vi "Flicker Main.vi"(8 "error in (no error)":errorcluster, 11 "Master":refnum<queue>) -> (0 "error out":errorcluster)   [LabVIEW 2014, in "Flicker.lvlib"]
doc: "This VI provides control and an interface for the photometric flicker measurements. It is built based on the queued message handler template and low level function VI's developed at CLTC. It is made to function as a stand-alone piece of sofware, or to be controlled by the Measurement Control package."
uses:
  Flicker.lvlib
  support/Message Queue/Message Cluster.ctl
  Settings/Settings.ctl
  Acquisition/Hardware Configuration.ctl
  Acquisition/Signal Type.ctl
  Logging/Logging Configuration.ctl
  controls/Flicker UI Data.ctl
  support/Message Queue/Enqueue Message (Single).vi
  support/Message Queue/Enqueue Message (Array).vi
  <vilib>/Utility/error.llb/Error Cluster From Error Code.vi
  <vilib>/ErrorRing/Error Ring.xnode
  Acquisition/Flicker Acquisition.lvlib
  Logging/Flicker Logging.lvlib
  Settings/Flicker Settings.lvlib
  support/User Event - Stop/Flicker User Event - Stop.lvlib
  support/Message Queue/Flicker Message Queue.lvlib
panel:
  out "Data":waveform(dbl)[](graph)
  in  "Settings":bool
  in  "Start Acquisition":bool
  in  "Stop":bool
  out "Status":string
  in  "Exit":bool
  # "Flicker"
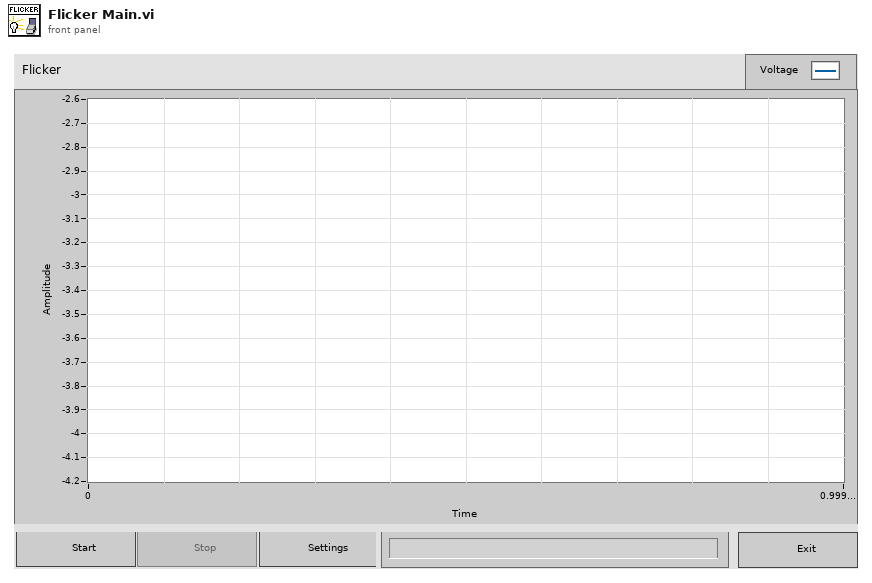
[diagram p1: front panel]
types:
  T1 = typedef "Flicker.lvlib/Flicker UI Data.ctl" = cluster{"Start Ref":refnum<vi>, "Stop Ref":refnum<vi>, "Settings Ref":refnum<vi>, "Exit Ref":refnum<vi>, "Status Ref":refnum<vi>, "WFGraph Refnum":refnum<vi>}
  T2 = typedef "Flicker.lvlib/Flicker Settings.lvlib/Settings.ctl" = cluster{"Hardware Configuration":T3, "Logging Configuration":T5}
  T3 = typedef "Flicker.lvlib/Flicker Acquisition.lvlib/Hardware Configuration.ctl" = cluster{"DAQmx Task Name":refnum<k21>, "HW Refnum <Replace Me>":string, "Signal Type <Replace Me>":T4}
  T4 = typedef "Flicker.lvlib/Flicker Acquisition.lvlib/Signal Type.ctl" = enum16{"Sine Wave", "Square with Noise"}
  T5 = typedef "Flicker.lvlib/Flicker Logging.lvlib/Logging Configuration.ctl" = cluster{"Log File Base Path":path, "TDMS File Reference":refnum<k34>}
  T6 = typedef "Flicker.lvlib/Flicker Message Queue.lvlib/All Message Queues.ctl" = cluster{"Master":refnum<queue>, "UI":refnum<queue>, "Acquisition":refnum<queue>, "Logging":refnum<queue>}
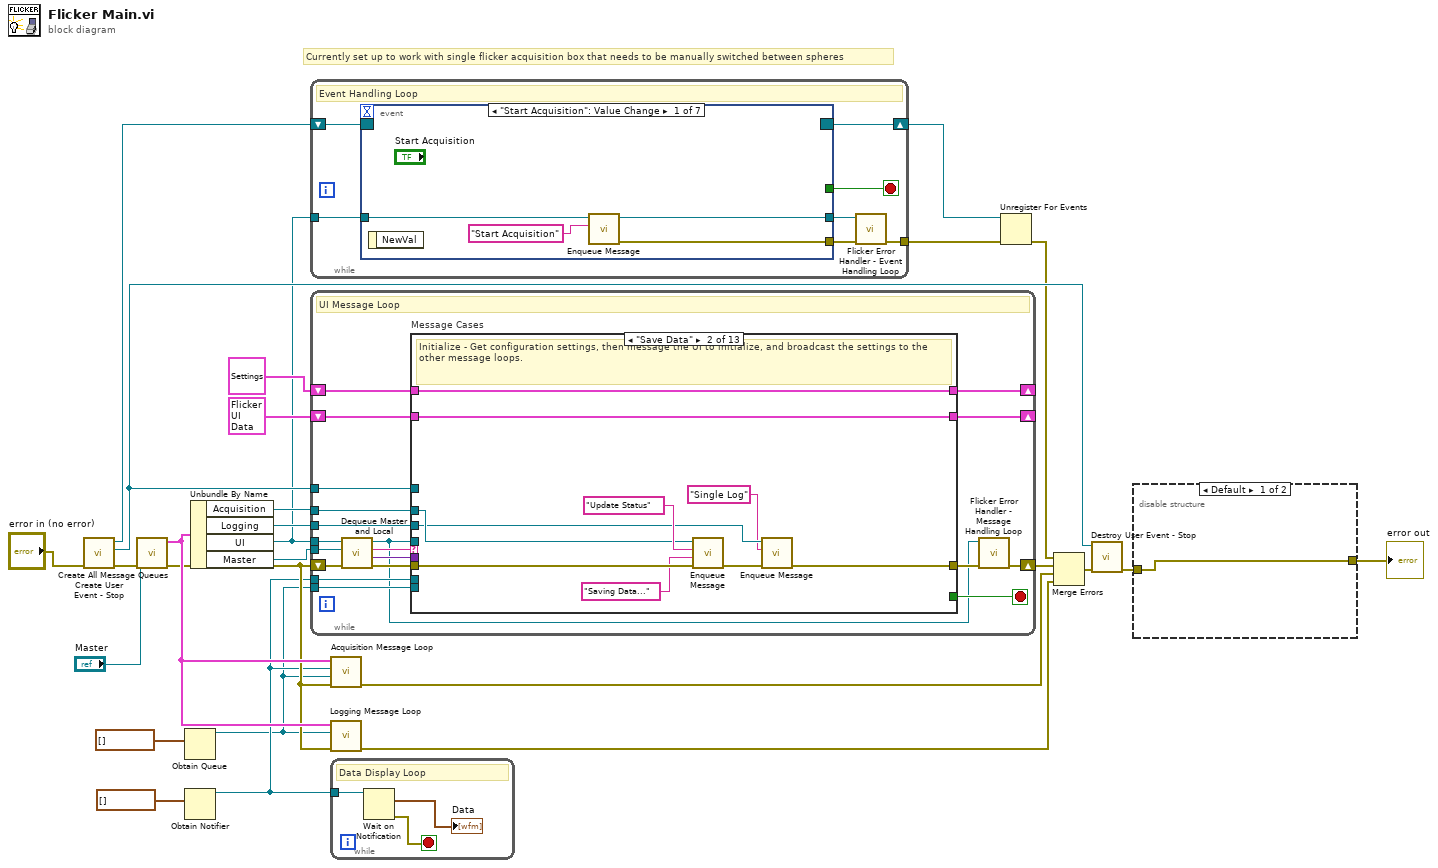
[diagram p0: block diagram]
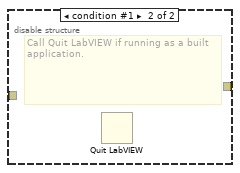
[diagram p2: hidden frame]
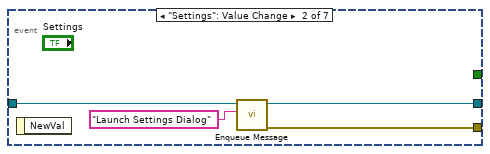
[diagram p3: hidden frame]
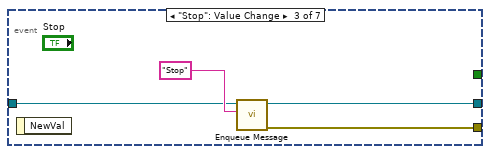
[diagram p4: hidden frame]
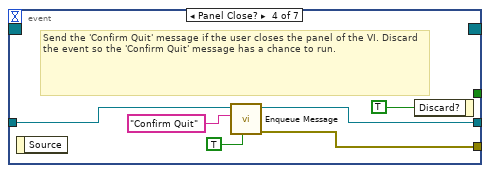
[diagram p5: hidden frame]
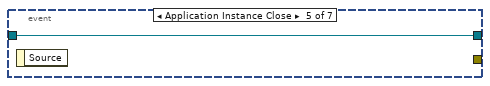
[diagram p6: hidden frame]
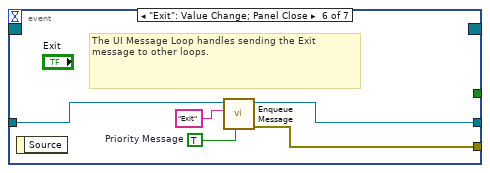
[diagram p7: hidden frame]
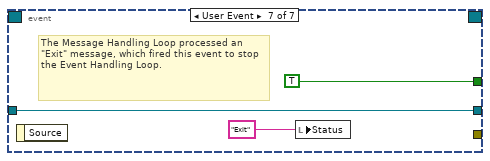
[diagram p8: hidden frame]
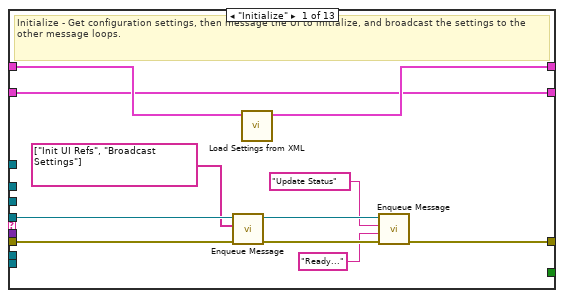
[diagram p9: hidden frame]
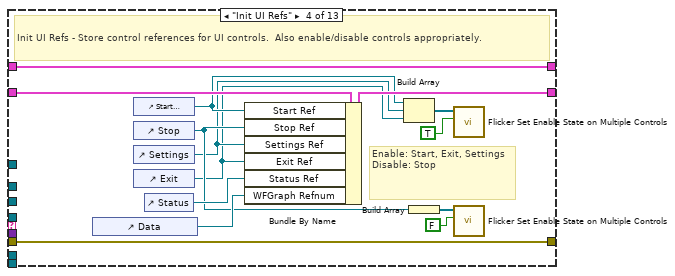
[diagram p11: hidden frame]
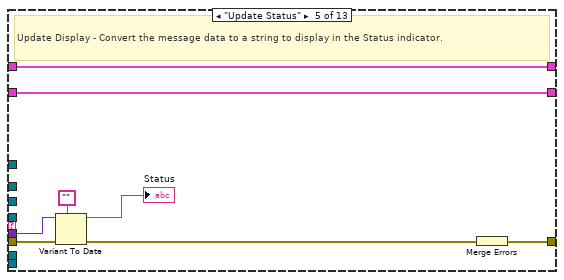
[diagram p12: hidden frame]
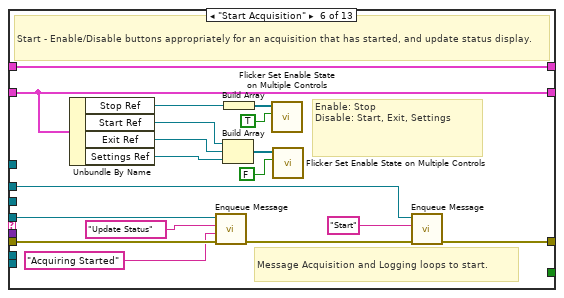
[diagram p13: hidden frame]
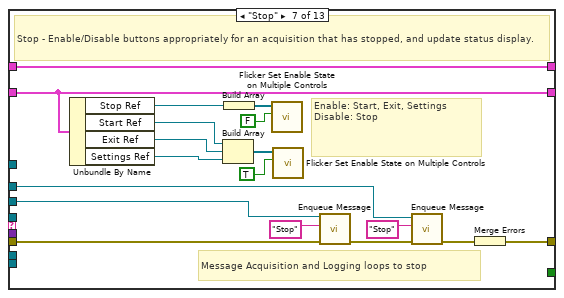
[diagram p14: hidden frame]
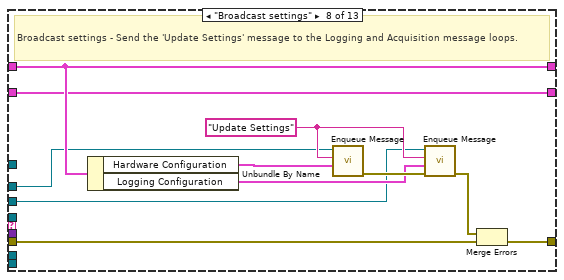
[diagram p15: hidden frame]
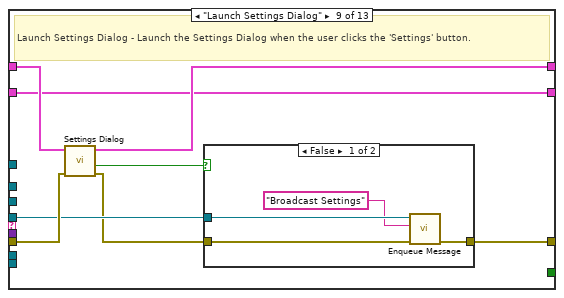
[diagram p16: hidden frame]
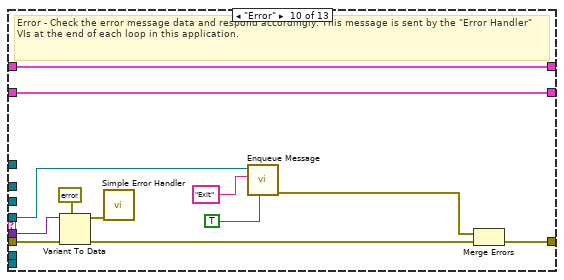
[diagram p18: hidden frame]
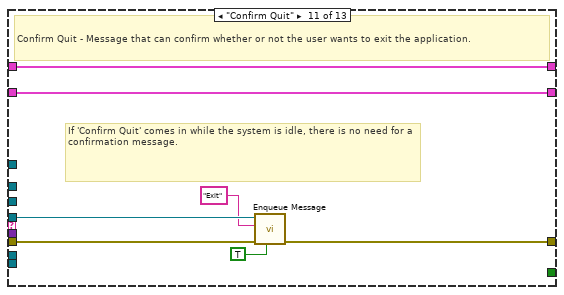
[diagram p19: hidden frame]
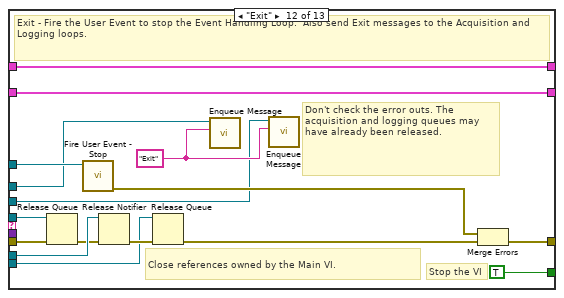
[diagram p20: hidden frame]
diagram:
  # "Currently set up to work with single flicker acquisition box that needs to be manually switched between spheres"
  n1 = call "Create User Event - Stop.vi"("error in (no error)"="error in (no error)") -> ("error out"=w21:errorcluster, "User Event - Stop"=w23:refnum<user-event>, "Stop Event Registration Refnum"=w24:refnum<event-registration>)  [unwired: 8 in]
  n2 = call "Create All Message Queues.vi"("error in (no error)"=w21, "Master Queue In"="Master") -> ("error out"=w18:errorcluster, "Message Queues out"=w20:T6)  [unwired: 8 in]
  n3 = Obtain Queue(element data type=waveform(dbl)[] []) -> (queue out=w7:refnum<queue>)  [unwired: 4 in, 2 out]
  n4 = Obtain Notifier(notification data type=waveform(dbl)[] []) -> (notifier out=w9:refnum<notifier>)  [unwired: 3 in, 2 out]
  n5 = Unbundle By Name(w20) -> ("Acquisition"=w13:refnum<queue>, "Logging"=w12:refnum<queue>, "UI"=w11:refnum<queue>, "Master"=w3:refnum<queue>)
  n6 = while {
    tunnel: w11 -> [w32]
    tunnel: [w29] -> w25
    shift-right: [w31] -> w15
    shift-left: w24 -> [w33]
    stop <- w30 stop-if-true
    # "Event Handling Loop"
    n7 = event shown="[0] \"Start Acquisition\": Value Change" {
      selector: w33 -> [_ _ _ _ _ _ _]
      dyn-events: [_ _ _ _ _ _ _] -> w31
      timeout: _ -> [_ _ _ _ _ _ _]
      tunnel: [_ _ _ _ _ _ TRUE ("Discard?")] -> w30
      tunnel: w32 -> [w37 w39 w44 w49 w52 w54 w58]
      tunnel: [w35 w41 w43 w47 _ w57 _] -> w28
      tunnel: [w34 w38 w42 w48 w52 w53 w58] -> w27
      event "Start Acquisition": Value Change {
        n8 = event-data() -> ()  [unwired: 1 in, 1 out]
        n9 = call-poly "Enqueue Message.vi"("Message"="Start Acquisition", "Message Queue"=w37) -> ("error out"=w35:errorcluster, "dup Message Queue"=w34:refnum<queue>)  [unwired: 8 in]
      }
      event "Settings": Value Change {
        n10 = event-data() -> ()  [unwired: 1 in, 1 out]
        n11 = call-poly "Enqueue Message.vi"("Message"="Launch Settings Dialog", "Message Queue"=w39) -> ("error out"=w41:errorcluster, "dup Message Queue"=w38:refnum<queue>)  [unwired: 8 in]
      }
      event "Stop": Value Change {
        n12 = event-data() -> ()  [unwired: 1 in, 1 out]
        n13 = call-poly "Enqueue Message.vi"("Message"="Stop", "Message Queue"=w44) -> ("error out"=w43:errorcluster, "dup Message Queue"=w42:refnum<queue>)  [unwired: 8 in]
      }
      event Panel Close? {
        # "Send the 'Confirm Quit' message if the user closes the panel of the VI. Discard the event so the 'Confirm Quit' message has a chance to run."
        n14 = event-data() -> ()  [unwired: 1 in, 1 out]
        n15 = call-poly "Enqueue Message.vi"("Priority Message? (F)"=TRUE, "Message"="Confirm Quit", "Message Queue"=w49) -> ("error out"=w47:errorcluster, "dup Message Queue"=w48:refnum<queue>)  [unwired: 7 in]
        n16 = event-data("Discard?"=TRUE) -> ()  [unwired: 1 in, 1 out]
      }
      event Application Instance Close {
        n17 = event-data() -> ()  [unwired: 1 in, 1 out]
      }
      event "Exit": Value Change; Panel Close {
        w55 = TRUE  # Priority Message
        # "The UI Message Loop handles sending the Exit message to other loops."
        n18 = event-data() -> ()  [unwired: 1 in, 1 out]
        n19 = call-poly "Enqueue Message.vi"("Priority Message? (F)"=w55, "Message"="Exit", "Message Queue"=w54) -> ("error out"=w57:errorcluster, "dup Message Queue"=w53:refnum<queue>)  [unwired: 7 in]
      }
      event User Event {
        # "The Message Handling Loop processed an \"Exit\" message, which fired this event to stop the Event Handling Loop."
        n20 = event-data() -> ()  [unwired: 1 in, 1 out]
        n21 = local write "Status"("Exit" ("Exit String")) -> ()
      }
    }
    n22 = call "Flicker Error Handler - Event Handling Loop.vi"("error in (no error)"=w28, "Message Queue"=w27) -> ("dup error in"=w29:errorcluster)  [unwired: 8 in, 1 out]
  }
  n23 = while {
    tunnel: w11 -> [w62]
    tunnel: w23 -> [w78]
    shift-right: [w69] -> w26
    shift-left: w18 -> [w63]
    shift-right: [w77] -> _
    shift-left: T2 {"Hardware Configuration"={"DAQmx Task Name"="", "HW Refnum <Replace Me>"="", "Signal Type <Replace Me>"=enum."Sine Wave"}, "Logging Configuration"={"Log File Base Path"=path "", "TDMS File Reference"=refnum}} ("Settings") -> [w76]
    shift-right: [w74] -> _
    shift-left: T1 {"Start Ref"=refnum, "Stop Ref"=refnum, "Settings Ref"=refnum, "Exit Ref"=refnum, "Status Ref"=refnum, "WFGraph Refnum"=refnum} ("Measurement UI Controls") -> [w75]
    tunnel: w13 -> [w73]
    tunnel: w12 -> [w72]
    tunnel: w9 -> [w71]
    tunnel: w7 -> [w70]
    tunnel: w3 -> [w61]
    stop <- w79 stop-if-true
    # "UI Message Loop"
    n24 = call "Dequeue Master and Local.vi"("error in (no error)"=w63, "Master Queue In"=w61, "UI In"=w62) -> ("error out"=w67:errorcluster, "Message Data"=w66:variant, "Message"=w65:string, "UI Out"=w64:refnum<queue>)  [unwired: 5 in]
    n25 = case "Message Cases" shown="\"Save Data\"" w65 {
      selector: w65 -> [_ _ _ _ _ _ _ _ _ _ _ _ w222]
      tunnel: w64 -> [w82 _ _ _ _ w143 _ _ w177 w190 w202 w210 _]
      tunnel: w67 -> [w81 w98 w101 w117 w124 w142 w160 w166 w179 w193 w201 w218 _]
      tunnel: [w86 w94 w101 w117 w125 w129 w161 w172 w174 w189 w200 w219 w221] -> w68
      tunnel: [_ _ _ _ _ _ _ _ _ _ _ TRUE _] -> w79
      tunnel: w66 -> [_ _ _ _ w123 _ _ _ _ w191 _ _ _]
      tunnel: w78 -> [_ _ _ _ _ _ _ _ _ _ _ w217 _]
      tunnel: [w89 w96 w102 w116 w119 w141 w159 w170 w176 w197 w204 w215 w224] -> w77
      tunnel: w76 -> [w90 w96 w102 w116 w119 w141 w159 w170 w180 w197 w204 w215 w224]
      tunnel: w75 -> [w83 w99 w103 w115 w118 w138 w158 w164 w173 w196 w203 w213 w223]
      tunnel: [w83 w99 w103 w112 w118 w138 w158 w164 w173 w196 w203 w213 w223] -> w74
      tunnel: w73 -> [_ w97 _ _ _ w128 w145 w163 _ _ _ w212 _]
      tunnel: w72 -> [_ w93 _ _ _ _ w148 w162 _ _ _ w211 _]
      tunnel: w71 -> [_ _ _ _ _ _ _ _ _ _ _ w209 _]
      tunnel: w70 -> [_ _ _ _ _ _ _ _ _ _ _ w205 _]
      frame "Initialize" {
        # "Initialize - Get configuration settings, then message the UI to initialize, and broadcast the settings to the other message loops."
        n26 = call-poly "Enqueue Message.vi"("error in (no error)"=w81, "Message Array"=string[] ["Init UI Refs", "Broadcast Settings"], "Message Queue"=w82) -> ("error out"=w88:errorcluster, "dup Message Queue"=w87:refnum<queue>)  [unwired: 7 in]
        n27 = call "Load Settings from XML.vi"("Settings in"=w90) -> ("Settings out"=w89:T2)  [unwired: 9 in, 1 out]
        n28 = call-poly "Enqueue Message.vi"("error in (no error)"=w88, "Message Data"="Ready..." ("Ready..."), "Message"="Update Status", "Message Queue"=w87) -> ("error out"=w86:errorcluster)  [unwired: 6 in, 1 out]
      }
      frame "Save Data" {
        # "Initialize - Get configuration settings, then message the UI to initialize, and broadcast the settings to the other message loops."
        n29 = call-poly "Enqueue Message.vi"("error in (no error)"=w98, "Message Data"="Saving Data..." ("Message"), "Message"="Update Status", "Message Queue"=w97) -> ("error out"=w95:errorcluster)  [unwired: 6 in, 1 out]
        n30 = call-poly "Enqueue Message.vi"("error in (no error)"=w95, "Message"="Single Log", "Message Queue"=w93) -> ("error out"=w94:errorcluster)  [unwired: 7 in, 1 out]
      }
      frame "Ignore Message" {
        # "Initialize - Get configuration settings, then message the UI to initialize, and broadcast the settings to the other message loops."
      }
      frame "Init UI Refs" {
        # "Enable: Start, Exit, Settings\nDisable: Stop"
        # "Init UI Refs - Store control references for UI controls.  Also enable/disable controls appropriately."
        n31 = control-ref of="Data"() -> (w113:refnum<vi>)
        n32 = control-ref of="Start Acquisition"() -> (w106:refnum<vi>)
        n33 = control-ref of="Stop"() -> (w107:refnum<vi>)
        n34 = control-ref of="Settings"() -> (w105:refnum<vi>)
        n35 = control-ref of="Exit"() -> (w104:refnum<vi>)
        n36 = control-ref of="Status"() -> (w114:refnum<vi>)
        n37 = Bundle By Name(cluster=w115, "Start Ref"=w106, "Stop Ref"=w107, "Settings Ref"=w105, "Exit Ref"=w104, "Status Ref"=w114, "WFGraph Refnum"=w113) -> (w112:T1)
        n38 = Build Array(w106, w105, w104) -> (w110:refnum<vi>[])
        n39 = Build Array(w107) -> (w109:refnum<vi>[])
        n40 = call "Flicker Set Enable State on Multiple Controls.vi"("Enable?"=TRUE, "Controls"=w110) -> ()  [unwired: 10 in]
        n41 = call "Flicker Set Enable State on Multiple Controls.vi"("Enable?"=FALSE, "Controls"=w109) -> ()  [unwired: 10 in]
      }
      frame "Update Status" {
        # "Update Display - Convert the message data to a string to display in the Status indicator."
        n42 = Variant To Data(error in=w124, type="", Variant=w123) -> (data=→"Status":string, error out=w121:errorcluster)
        n43 = Merge Errors(w121) -> (w125:errorcluster)
      }
      frame "Start Acquisition" {
        # "Message Acquisition and Logging loops to start."
        # "Enable: Stop\nDisable: Start, Exit, Settings"
        # "Start - Enable/Disable buttons appropriately for an acquisition that has started, and update status display."
        n44 = Unbundle By Name(w138) -> ("Stop Ref"=w133:refnum<vi>, "Start Ref"=w132:refnum<vi>, "Exit Ref"=w131:refnum<vi>, "Settings Ref"=w130:refnum<vi>)
        n45 = call-poly "Enqueue Message.vi"("error in (no error)"=w142, "Message Data"="Acquiring Started" ("Acquiring and Logging..."), "Message"="Update Status", "Message Queue"=w143) -> ("error out"=w126:errorcluster)  [unwired: 6 in, 1 out]
        n46 = Build Array(w132, w131, w130) -> (w136:refnum<vi>[])
        n47 = Build Array(w133) -> (w135:refnum<vi>[])
        n48 = call "Flicker Set Enable State on Multiple Controls.vi"("Enable?"=TRUE, "Controls"=w135) -> ()  [unwired: 10 in]
        n49 = call "Flicker Set Enable State on Multiple Controls.vi"("Enable?"=FALSE, "Controls"=w136) -> ()  [unwired: 10 in]
        n50 = call-poly "Enqueue Message.vi"("error in (no error)"=w126, "Message"="Start", "Message Queue"=w128) -> ("error out"=w129:errorcluster)  [unwired: 7 in, 1 out]
      }
      frame "Stop" {
        # "Message Acquisition and Logging loops to stop"
        # "Enable: Start, Exit, Settings\nDisable: Stop"
        # "Stop - Enable/Disable buttons appropriately for an acquisition that has stopped, and update status display."
        n51 = Unbundle By Name(w158) -> ("Stop Ref"=w153:refnum<vi>, "Start Ref"=w152:refnum<vi>, "Exit Ref"=w151:refnum<vi>, "Settings Ref"=w150:refnum<vi>)
        n52 = Build Array(w152, w151, w150) -> (w156:refnum<vi>[])
        n53 = Build Array(w153) -> (w155:refnum<vi>[])
        n54 = call "Flicker Set Enable State on Multiple Controls.vi"("Enable?"=FALSE, "Controls"=w155) -> ()  [unwired: 10 in]
        n55 = call "Flicker Set Enable State on Multiple Controls.vi"("Enable?"=TRUE, "Controls"=w156) -> ()  [unwired: 10 in]
        n56 = call-poly "Enqueue Message.vi"("error in (no error)"=w160, "Message"="Stop", "Message Queue"=w148) -> ("error out"=w147:errorcluster)  [unwired: 7 in, 1 out]
        n57 = call-poly "Enqueue Message.vi"("error in (no error)"=w147, "Message"="Stop", "Message Queue"=w145) -> ("error out"=w146:errorcluster)  [unwired: 7 in, 1 out]
        n58 = Merge Errors(w146) -> (w161:errorcluster)
      }
      frame "Broadcast settings" {
        w165 = "Update Settings" ("Message")
        # "Broadcast settings - Send the 'Update Settings' message to the Logging and Acquisition message loops."
        n59 = Unbundle By Name(w170) -> ("Hardware Configuration"=w169:T3, "Logging Configuration"=w168:T5)
        n60 = call-poly "Enqueue Message.vi"("Message Data"=w169, "Message"=w165, "Message Queue"=w163) -> ("error out"=w171:errorcluster)  [unwired: 7 in, 1 out]
        n61 = call-poly "Enqueue Message.vi"("error in (no error)"=w171, "Message Data"=w168, "Message"=w165, "Message Queue"=w162) -> ("error out"=w167:errorcluster)  [unwired: 6 in, 1 out]
        n62 = Merge Errors(w167, w166) -> (w172:errorcluster)
      }
      frame "Launch Settings Dialog" {
        # "Launch Settings Dialog - Launch the Settings Dialog when the user clicks the 'Settings' button."
        n63 = call "Settings Dialog.vi"("error in (no error)"=w179, "Settings in"=w180) -> ("error out"=w175:errorcluster, "Cancelled?"=w178:bool, "Settings out"=w176:T2)  [unwired: 6 in, 1 out]
        n64 = case shown="False" w178 {
          tunnel: w177 -> [w184 _]
          tunnel: w175 -> [w183 w185]
          tunnel: [w182 w185] -> w174
          frame False {
            n65 = call-poly "Enqueue Message.vi"("error in (no error)"=w183, "Message"="Broadcast Settings", "Message Queue"=w184) -> ("error out"=w182:errorcluster)  [unwired: 7 in, 1 out]
          }
          frame True {
          }
        }
      }
      frame "Error" {
        # "Error - Check the error message data and respond accordingly. This message is sent by the \"Error Handler\" VIs at the end of each loop in this application."
        n66 = Variant To Data(error in=w193, type=errorcluster {"status"=FALSE, "code"=0, "source"=""} ("error constant"), Variant=w191) -> (data=w195:errorcluster, error out=w192:errorcluster)
        n67 = call <vilib>:"Simple Error Handler.vi"("error in (no error)"=w195) -> ()  [unwired: 4 in, 5 out]
        n68 = call-poly "Enqueue Message.vi"("Priority Message? (F)"=TRUE, "Message"="Exit", "Message Queue"=w190) -> ("error out"=w188:errorcluster)  [unwired: 7 in, 1 out]
        n69 = Merge Errors(w188, w192) -> (w189:errorcluster)
      }
      frame "Confirm Quit" {
        # "If 'Confirm Quit' comes in while the system is idle, there is no need for a confirmation message."
        # "Confirm Quit - Message that can confirm whether or not the user wants to exit the application."
        n70 = call-poly "Enqueue Message.vi"("Priority Message? (F)"=TRUE, "error in (no error)"=w201, "Message"="Exit", "Message Queue"=w202) -> ("error out"=w200:errorcluster)  [unwired: 6 in, 1 out]
      }
      frame "Exit" {
        w214 = "Exit" ("Message")
        # "Don't check the error outs. The acquisition and logging queues may have already been released."
        # "Close references owned by the Main VI."
        # "Stop the VI"
        # "Exit - Fire the User Event to stop the Event Handling Loop.  Also send Exit messages to the Acquisition and Logging loops."
        n71 = Release Queue(queue=w210, error in (no error)=w218) -> (error out=w208:errorcluster)  [unwired: 1 in, 2 out]
        n72 = call "Fire User Event - Stop.vi"("User Event - Stop"=w217) -> ("error out"=w216:errorcluster)  [unwired: 10 in]
        n73 = Release Notifier(notifier=w209, error in (no error)=w208) -> (error out=w207:errorcluster)  [unwired: 1 in, 2 out]
        n74 = Release Queue(queue=w205, error in (no error)=w207) -> (error out=w206:errorcluster)  [unwired: 1 in, 2 out]
        n75 = call-poly "Enqueue Message.vi"("Message"=w214, "Message Queue"=w212) -> ()  [unwired: 8 in, 2 out]
        n76 = call-poly "Enqueue Message.vi"("Message"=w214, "Message Queue"=w211) -> ()  [unwired: 8 in, 2 out]
        n77 = Merge Errors(w216, w206) -> (w219:errorcluster)
      }
      frame Default {
        # "'Default' case only runs if there is a message that isn't defined in any of the other cases.  Output a programming error."
        n78 = xnode "Error Ring"("parameter 0"=w222) -> ("error out"=w221:errorcluster)
      }
    }
    n79 = call "Flicker Error Handler - Message Handling Loop.vi"("error in (no error)"=w68, "Message Queue"=w64) -> ("dup error in"=w69:errorcluster)  [unwired: 8 in, 1 out]
  }
  n80 = call "Acquisition Message Loop.vi"("error in (no error)"=w18, "Data Queue"=w7, "Data Notifier"=w9, "Message Queues"=w20) -> ("error out"=w22:errorcluster)  [unwired: 7 in]
  n81 = call "Logging Message Loop.vi"("error in (no error)"=w18, "Data Queue"=w7, "Message Queues"=w20) -> ("error out"=w19:errorcluster)  [unwired: 8 in]
  n82 = while "Data Display Loop" {
    tunnel: w9 -> [w234]
    stop <- w232 stop-if-true
    # "Data Display Loop"
    n83 = Wait on Notification(notifier=w234) -> (notification=→"Data":waveform(dbl)[], error out=w232:errorcluster)  [unwired: 3 in, 2 out]
  }
  n84 = Unregister For Events(event registration refnum=w15, error in=w25) -> (error out=w16:errorcluster)
  n85 = Merge Errors(w16, w26, w22, w19) -> (w5:errorcluster)
  n86 = call "Destroy User Event - Stop.vi"("error in (no error)"=w5, "User Event - Stop"=w23) -> ("error out"=w6:errorcluster)  [unwired: 9 in]
  n87 = disable-structure shown="Default" {
    disable-tunnel: w6 -> [w235 _]
    disable-tunnel: [w235 _] -> w2
    frame condition #0 (active) {
    }
    frame condition #1 {
      # "Call Quit LabVIEW if running as a built application."
      n88 = Quit LabVIEW() -> ()  [unwired: 1 in]
    }
  }
  "error out" <- w2
